vi "RhodeSchwarz_write_all_to_tdms.vi"(6 "timestamp":dbl format="%#_13g", 8 "error in (no error)":errorcluster, 9 "wfm info":T1(array[cluster]), 10 "Scaled Waveform":waveform(dbl)[](array[waveform]), 11 "file path":path) -> (0 "error out":errorcluster)   [LabVIEW 2020, in "RohdeSchwarz_RTA4000.lvclass"]
uses:
  RohdeSchwarz_RTA4000.lvclass
  shared/OnOffTypeDef.ctl
  <userlib>/_OpenG.lib/file/file.llb/Strip Path Extension - Path__ogtk.vi
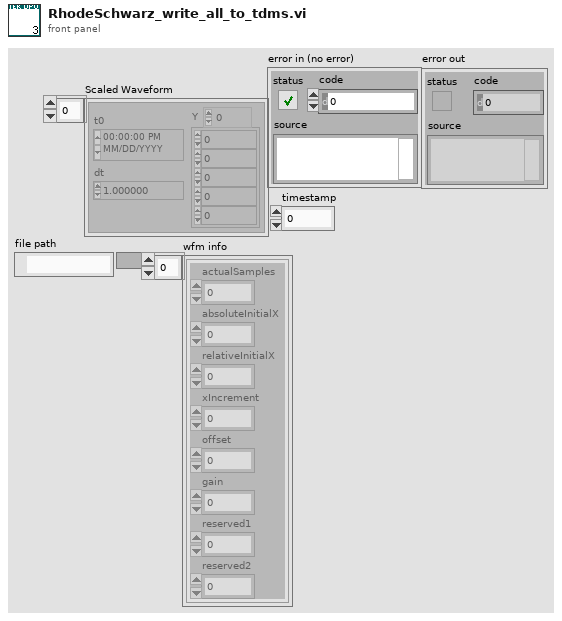
[diagram p1: front panel]
types:
  T1 = cluster{"actualSamples":i32, "absoluteInitialX":dbl, "relativeInitialX":dbl, "xIncrement":dbl, "offset":dbl, "gain":dbl, "reserved1":dbl, "reserved2":dbl}[]
  T2 = typedef "OnOffTypeDef.ctl" = enum16{"off", "on"}
  T3 = enum16{"open", "open or create", "create or replace", "create", "open (read-only)"}
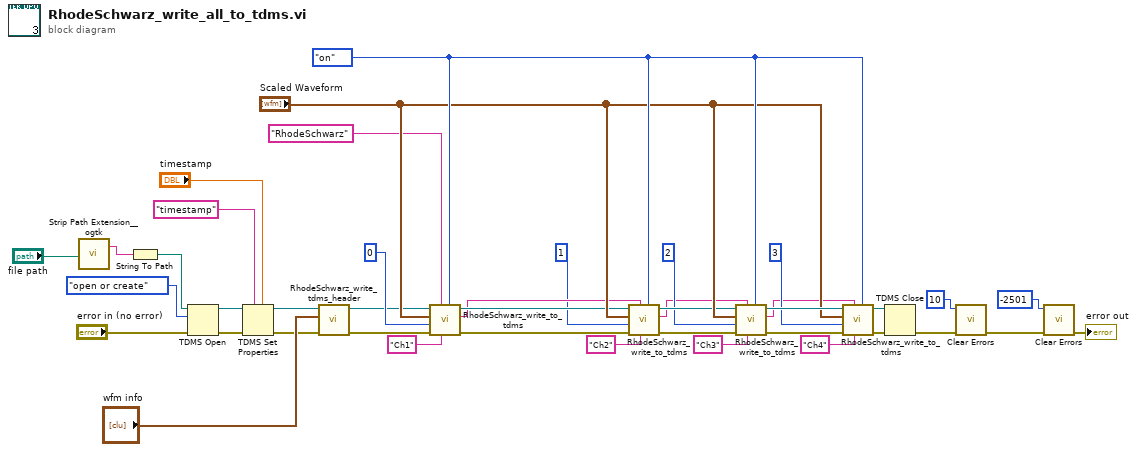
[diagram p0: block diagram]
diagram:
  w38 = OnOffTypeDef."on" ("EnableChA")
  n1 = call-poly <userlib>:"Strip Path Extension__ogtk.vi"("path"="file path") -> ("root"=w2:string)  [unwired: 1 out]
  n2 = String To Path(string=w2) -> (path=w1:path)
  n3 = TDMS Open(8:"error in (no error)", 10:T3."open or create" ("operation"), 11:w1) -> (0:w19:errorcluster, 3:w20:refnum<k34>)  [unwired: 4 in]
  n4 = TDMS Set Properties(5:"timestamp", 7:"timestamp", 8:w19, 11:w20) -> (0:w5:errorcluster, 3:w7:refnum<k34>)  [unwired: 2 in, 2 out]
  n5 = call "RhodeSchwarz_write_tdms_header.vi"("error in (no error)"=w5, "wfm info"="wfm info", "Refnum in"=w7) -> ("error out"=w4:errorcluster, "Refnum out"=w6:refnum<k34>)  [unwired: 7 in]
  n6 = call "RhodeSchwarz_write_to_tdms.vi"("EnableChA"=w38, "channel name"="Ch1", "group name in (Untitled)"="RhodeSchwarz", "error in (no error)"=w4, "index"=0, "ScopeTraces"="Scaled Waveform", "Refnum in"=w6) -> ("error out"=w24:errorcluster, "group name out"=w26:string, "Refnum out"=w27:refnum<k34>)  [unwired: 2 in]
  n7 = call "RhodeSchwarz_write_to_tdms.vi"("EnableChA"=w38, "channel name"="Ch2", "group name in (Untitled)"=w26, "error in (no error)"=w24, "index"=1, "ScopeTraces"="Scaled Waveform", "Refnum in"=w27) -> ("error out"=w30:errorcluster, "group name out"=w11:string, "Refnum out"=w32:refnum<k34>)  [unwired: 2 in]
  n8 = call "RhodeSchwarz_write_to_tdms.vi"("EnableChA"=w38, "channel name"="Ch3", "group name in (Untitled)"=w11, "error in (no error)"=w30, "index"=2, "ScopeTraces"="Scaled Waveform", "Refnum in"=w32) -> ("error out"=w34:errorcluster, "group name out"=w9:string, "Refnum out"=w36:refnum<k34>)  [unwired: 2 in]
  n9 = call "RhodeSchwarz_write_to_tdms.vi"("EnableChA"=w38, "channel name"="Ch4", "group name in (Untitled)"=w9, "error in (no error)"=w34, "index"=3, "ScopeTraces"="Scaled Waveform", "Refnum in"=w36) -> ("error out"=w40:errorcluster, "Refnum out"=w39:refnum<k34>)  [unwired: 2 in, 1 out]
  n10 = TDMS Close(8:w40, 11:w39) -> (0:w18:errorcluster)  [unwired: 1 out]
  n11 = call <vilib>:"Clear Errors.vi"("error in (no error)"=w18, "specific error code to clear (0: all)"=10) -> ("error out"=w16:errorcluster)  [unwired: 4 in, 1 out]
  n12 = call <vilib>:"Clear Errors.vi"("error in (no error)"=w16, "specific error code to clear (0: all)"=-2501) -> ("error out"=→"error out":errorcluster)  [unwired: 4 in, 1 out]
